vi "imagenesss.vi"() -> ()   [LabVIEW 2020]
panel:
  in  "Tab Control":T1(tab)
  in  "Method response":string
  in  "N/A":bool
  out "Conneted ?":bool
  in  "Password":string
  in  "Remote\n(Hostname or IPAddress":string
  in  "User":string
  in  "Password":string
  in  "OK Button 3":bool
  in  "OK Button 4":bool
  in  "RTU BaudRate":string(combo)
  in  "RTU  Parity":string(combo)
  in  "Channel(0)":bool
  in  "Channel(1)":bool
  in  "Channel(2)":bool
  in  "OK Button 5":bool
  in  "OK Button 6":bool
  in  "SSID":string
  in  "Wifi Password":string
  in  "Wifi IP Address":string
  in  "Wifi router":string
  out "Dynamic IP":bool
  in  "WLAN Priority":string(combo)
  in  "Ethernet IP Address":string
  in  "Ethernet router":string
  out "Dynamic IP":bool
  in  "LAN Priority":string(combo)
  in  "APN":string
  in  "Default Modem Device":string(combo)
  in  "OK Button":bool
  in  "OK Button 2":bool
  in  "stop":bool
  # "Unlock advanced settings"
  # "AC channels adjustment"
  # "DC Channels:"
  # "Wife Connection"
  # "Ethernet Connection"
  # "Cellular Connection (High priority)"
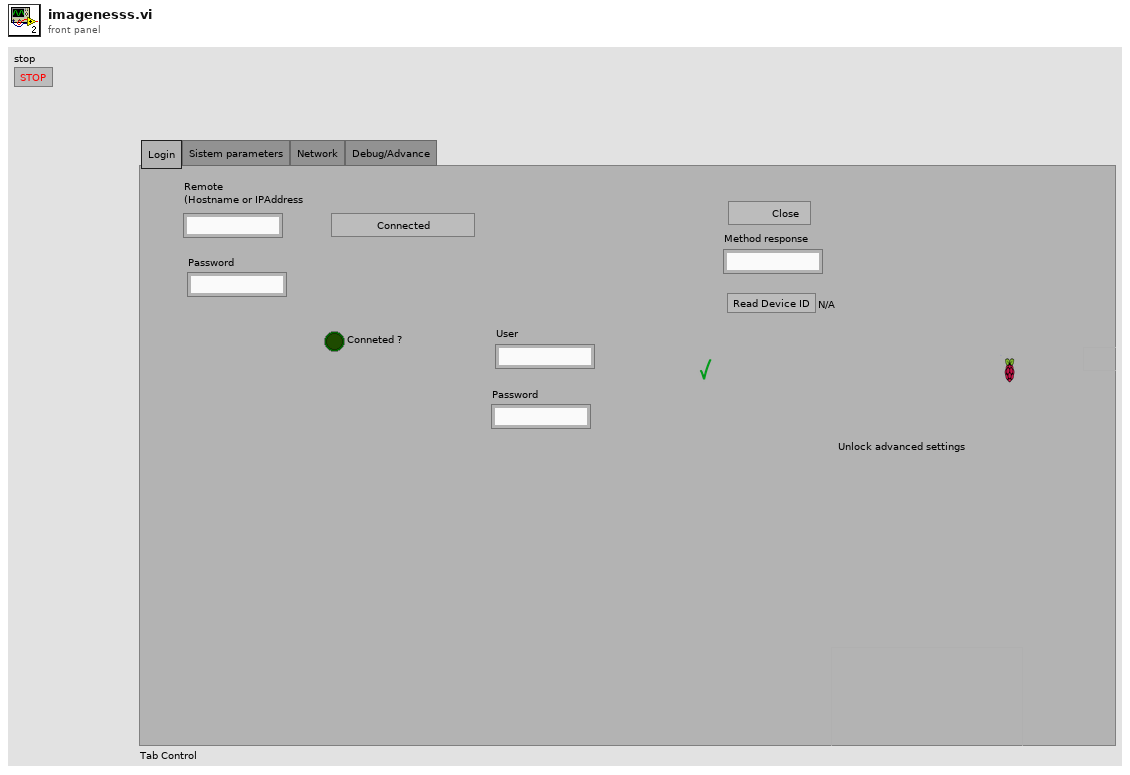
[diagram p1: front panel]
types:
  T1 = enum32{"Login", "Sistem parameters", "Network", "Debug/Advance"}
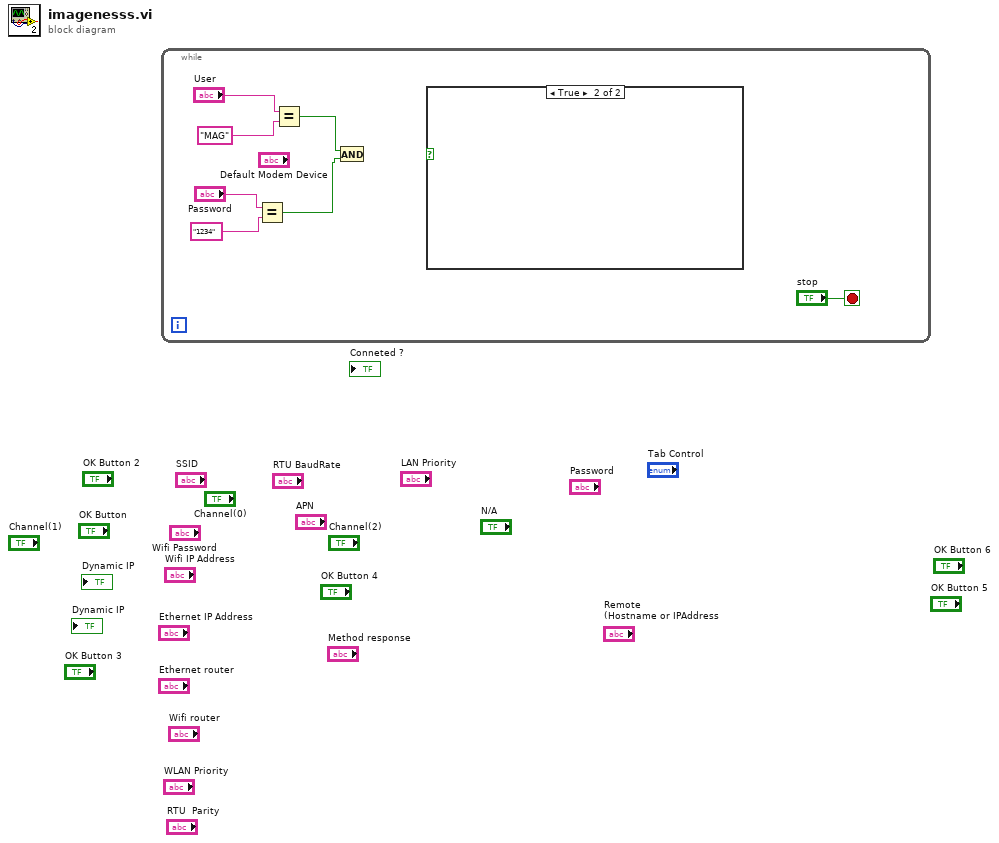
[diagram p0: block diagram]
diagram:
  n1 = while {
    stop <- "stop" stop-if-true
    n2 = Equal?(x="Password", y="1234") -> (x = y?=w1:bool)
    n3 = Equal?(x="User", y="MAG") -> (x = y?=w2:bool)
    n4 = And(x=w2, y=w1) -> ()  [unwired: 1 out]
    n5 = case shown="True" {
      selector: _ -> [_ _]
      frame False {
      }
      frame True {
      }
    }
  }
